vi "Write Settings.vi"(8 "error in (no error)":errorcluster, 10 "Dot Settings.lvclass":refnum<class "Dot Settings.lvclass">, 11 "Tool Dots in":refnum<class "Tool Dots.lvclass">) -> (0 "error out":errorcluster, 3 "Tool Dots out":refnum<class "Tool Dots.lvclass">)   [LabVIEW 2019, in "Tool Dots.lvclass"]
uses:
  Tool Dots.lvclass
  Settings/Dot Settings/Dot Settings.lvclass
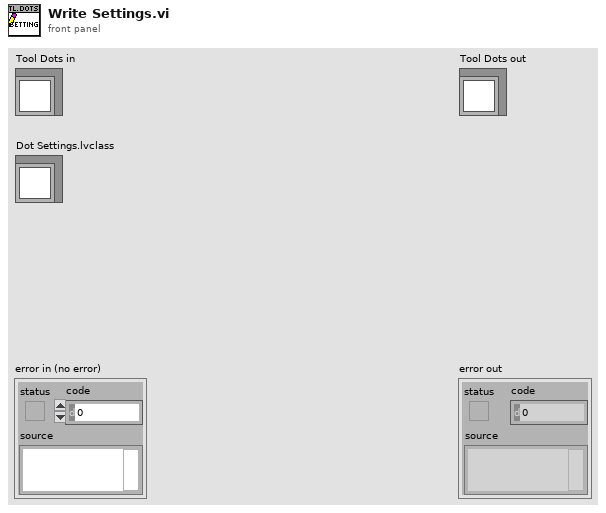
[diagram p1: front panel]
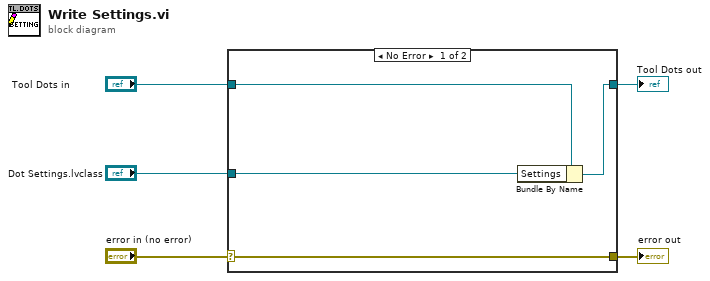
[diagram p0: block diagram]
diagram:
  n1 = case shown="No Error" "error in (no error)" {
    selector: "error in (no error)" -> [w9 w10]
    tunnel: [w9 w10] -> w4
    tunnel: [w7 w11] -> w2
    tunnel: "Tool Dots in" -> [w8 w11]
    tunnel: "Dot Settings.lvclass" -> [w6 _]
    frame No Error {
      n2 = Bundle By Name(cluster=w8, "Settings"=w6) -> (w7:refnum<class "Tool Dots.lvclass">)
    }
    frame Error {
    }
  }
  "error out" <- w4
  "Tool Dots out" <- w2
